vi "macro_LeadLag.vi"   [LabVIEW 2019, in "Trajectory_Library.lvlib"]
uses:
  Trajectory_Library.lvlib
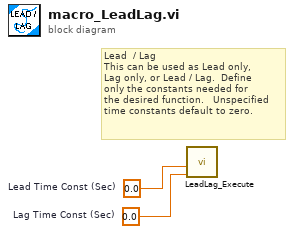
[diagram p0: block diagram]
diagram:
  w1 = 0.0  # Lag Time Const (Sec)
  w2 = 0.0  # Lead Time Const (Sec)
  # "Lead  / Lag\nThis can be used as Lead only, \nLag only, or Lead / Lag.  Define\nonly the constants needed for \nthe desired function.   Unspecified\ntime constants default to zero."
  n1 = call "LeadLag_Execute.vi"("Lag Time Const (Sec)"=w1, "Lead Time Const (Sec)"=w2) -> ()  [unwired: 9 in, 1 out]
